vi "Read Trace Buffer.vi"(8 "error in (no error)":errorcluster, 11 "VISA resource name":refnum<visa-resource-name>) -> (0 "error out":errorcluster, 1 "Reserved Size":i32, 2 "Total Size":i32, 3 "VISA resource name out":refnum<visa-resource-name>, 5 "Actual Trace Buffer Size":i32=1)   [LabVIEW 2020, in "Keithley 6517.lvlib"]
doc: "Returns the number of bytes of memory available, number of bytes reserved to store readings and the number of readings in the trace buffer."
uses:
  <instrlib>/Keithley 6517/Keithley 6517.lvlib
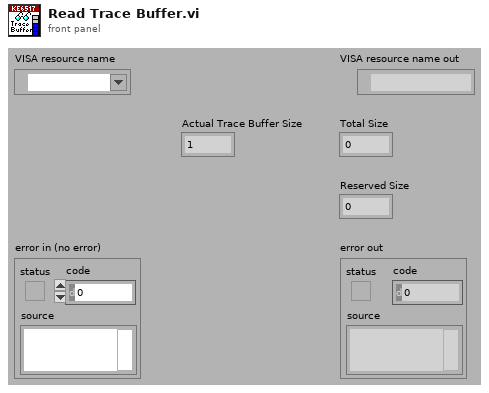
[diagram p1: front panel]
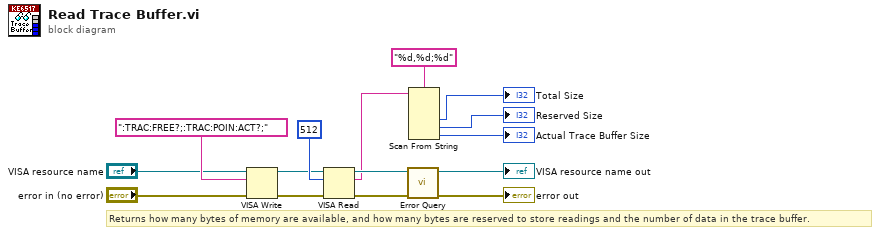
[diagram p0: block diagram]
diagram:
  # "Returns how many bytes of memory are available, and how many bytes are reserved to store readings and the number of data in the trace buffer."
  n1 = VISA Write(VISA resource name="VISA resource name", write buffer=":TRAC:FREE?;:TRAC:POIN:ACT?;", error in (no error)="error in (no error)") -> (VISA resource name out=w11:refnum<visa-resource-name>, error out=w10:errorcluster)  [unwired: 1 out]
  n2 = VISA Read(VISA resource name=w11, byte count=u32 512, error in (no error)=w10) -> (VISA resource name out=w9:refnum<visa-resource-name>, read buffer=w7:string, error out=w8:errorcluster)  [unwired: 1 out]
  n3 = call <instrlib>:"Error Query.vi"("error in (no error)"=w8, "VISA resource name"=w9) -> ("error out"=→"error out":errorcluster, "VISA resource name out"=→"VISA resource name out":refnum<visa-resource-name>)  [unwired: 6 in, 2 out]
  n4 = Scan From String(format string="%d,%d;%d", input string=w7) -> (output 1=→"Total Size":i32, output 2=→"Reserved Size":i32, output 3=→"Actual Trace Buffer Size":i32)  [unwired: 5 in, 3 out]
